vi "Get Project Library Suffix.vi"(8 "error in (no error)":errorcluster) -> (0 "error out":errorcluster, 2 "Project Library Suffix":string)   [LabVIEW 2017, in "Test Explorer.lvlib"]
doc: "Returns the project library suffix defined in the settings file or default if undefined."
uses:
  Test Explorer.lvlib
  Configuration/Configuration.lvlib
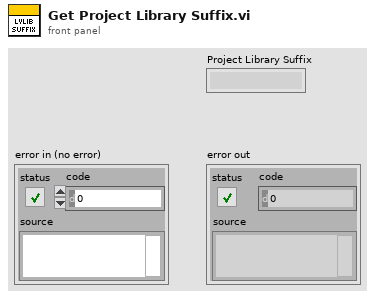
[diagram p1: front panel]
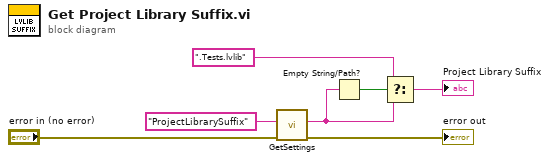
[diagram p0: block diagram]
diagram:
  n1 = call "GetSettings.vi"("error in (no error)"="error in (no error)", "Name"="ProjectLibrarySuffix") -> ("error out"=→"error out":errorcluster, "Value"=w5:string)  [unwired: 8 in]
  n2 = Empty String/Path?(string/path=w5) -> (empty?=w6:bool)
  n3 = Select(t=".Tests.lvlib" ("regular expression"), s=w6, f=w5) -> (s? t:f=→"Project Library Suffix":string)
